vi "VISA Port selector.vi"(1 "Defualt":refnum<visa-resource-name>, 2 "I/P":refnum<visa-resource-name>) -> (0 "O/P":refnum<visa-resource-name>)   [LabVIEW 2015]
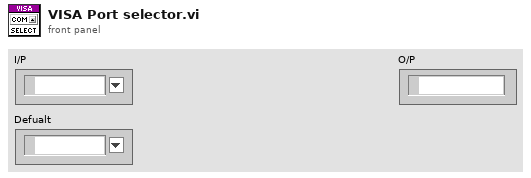
[diagram p1: front panel]
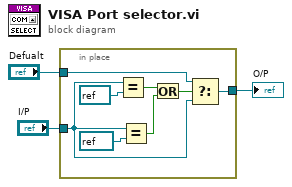
[diagram p0: block diagram]
diagram:
  n1 = in-place {
    in-place-border: "I/P" -> [w5]
    in-place-border: "Defualt" -> [w6]
    in-place-border: [w4] -> w1
    n2 = Equal?(x=w5, y=refnum<visa-resource-name> " " ("I/P")) -> (x = y?=w9:bool)
    n3 = Equal?(x=w5, y=refnum<visa-resource-name> refnum ("I/P")) -> (x = y?=w8:bool)
    n4 = Or(x=w9, y=w8) -> (x .or. y?=w7:bool)
    n5 = Select(t=w6, s=w7, f=w5) -> (s? t:f=w4:refnum<visa-resource-name>)
  }
  "O/P" <- w1
